vi "refocusAndReposition.vi"() -> ()   [LabVIEW 2022 SP3]
panel:
  in  "Point of Interest - y":dbl
  in  "Point of Interest - x":dbl
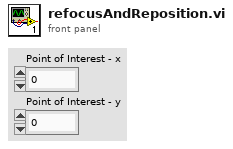
[diagram p1: front panel]
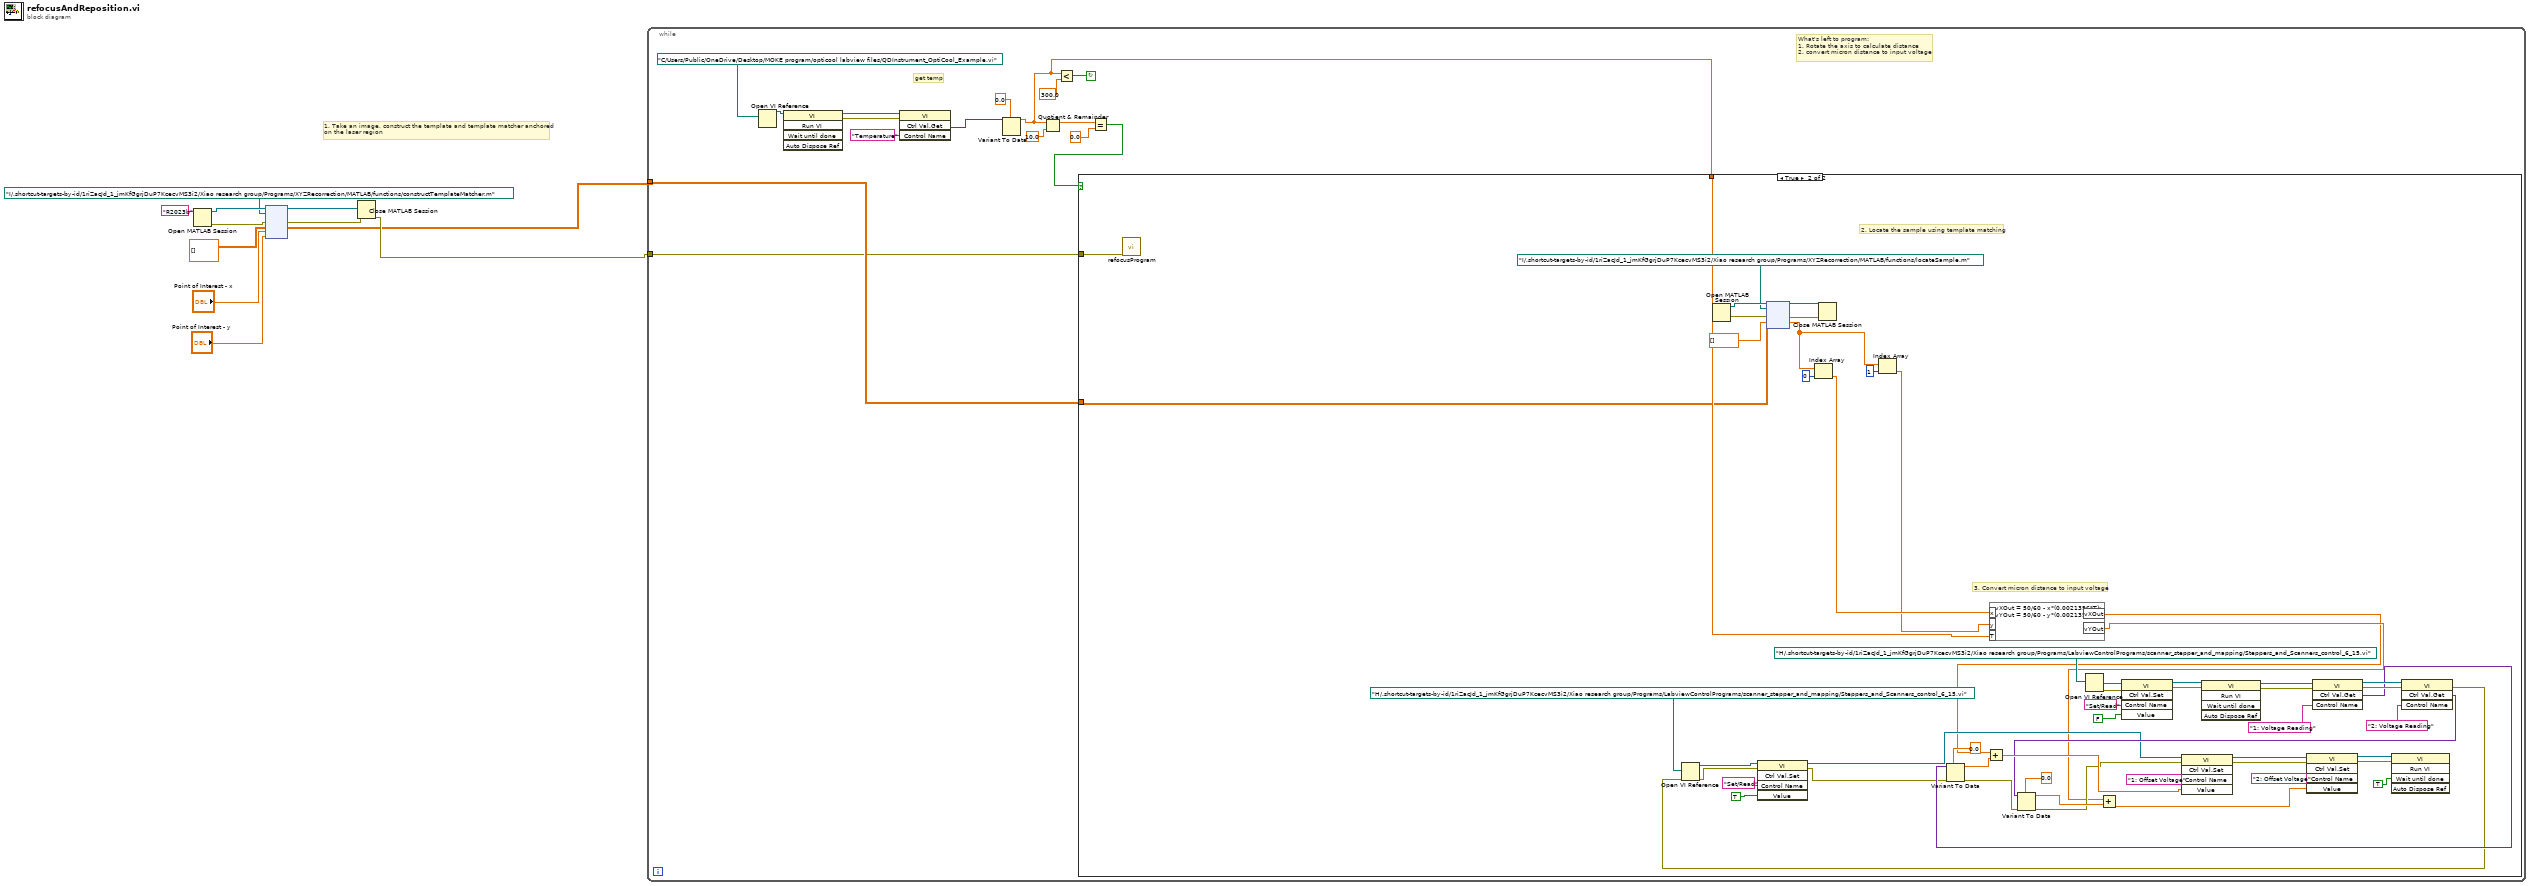
[diagram p0: block diagram]
diagram:
  # "1. Take an image, construct the template and template matcher anchored\non the laser region"
  n1 = Open MATLAB Session(0:"R2023b" ("release name")) -> (8:w11:refnum<k37>, 11:w10:errorcluster)  [unwired: 1 in]
  n2 = node(w11, path "I:/.shortcut-targets-by-id/1riZacJd_1_jmKfGgrjDuP7KcecvMS3i2/Xiao research group/Programs/XYZRecorrection/MATLAB/functions/constructTemplateMatcher.m" ("source file path"), w10, dbl[][] [], "Point of Interest - x", "Point of Interest - y") -> (w5:refnum<k37>, w4:errorcluster, w1:dbl[][])  [unwired: 3 in, 2 out]
  n3 = Close MATLAB Session(0:w5, 3:w4) -> (11:w2:errorcluster)
  n4 = while {
    tunnel: w1 -> [w14]
    tunnel: w2 -> [w13]
    stop <- w20 continue-if-true
    # "get temp"
    # "What's left to program:\n1. Rotate the axis to calculate distance\n2. convert micron distance to input voltage"
    n5 = Open VI Reference(vi path=path "C:/Users/Public/OneDrive/Desktop/MOKE program/opticool labview files/QDInstrument_OptiCool_Example.vi") -> (vi reference=w24:refnum<vi>)  [unwired: 5 in, 1 out]
    n6 = invoke class="VI" method="Run VI"(reference=w24) -> (reference out=w25:refnum<vi>, error out=w26:errorcluster)  [unwired: 4 in, 3 out]
    n7 = invoke class="VI" method="Ctrl Val.Get"(reference=w25, error in=w26, "Control Name"="Temperature") -> ("Get Control Value Variant"=w27:variant)  [unwired: 1 in, 3 out]
    n8 = Variant To Data(type=0.0, Variant=w27) -> (data=w12:dbl)  [unwired: 1 in, 1 out]
    n9 = Quotient & Remainder(x=w12, y=10.0) -> (x-y*floor(x/y)=w17:dbl)  [unwired: 1 out]
    n10 = Less?(x=w12, y=300.0) -> (x < y?=w20:bool)
    n11 = Equal?(x=w17, y=0.0) -> (x = y?=w15:bool)
    n12 = case shown="True" w15 {
      tunnel: w14 -> [_ w70]
      tunnel: w13 -> [_ w81]
      tunnel: w12 -> [_ w80]
      frame False {
      }
      frame True {
        # "3. Convert micron distance to input voltage"
        # "2. Locate the sample using template matching"
        n13 = call "refocusProgram.vi"("error in (no error)"=w81) -> ()  [unwired: 11 in]
        n14 = Open MATLAB Session() -> (8:w79:refnum<k37>, 11:w76:errorcluster)  [unwired: 2 in]
        n15 = node(w79, path "I:/.shortcut-targets-by-id/1riZacJd_1_jmKfGgrjDuP7KcecvMS3i2/Xiao research group/Programs/XYZRecorrection/MATLAB/functions/locateSample.m" ("source file path"), w76, dbl[] [], w70) -> (w78:refnum<k37>, w77:errorcluster, w72:dbl[])  [unwired: 2 in, 2 out]
        n16 = Index Array(array=w72, index=0 ("index (row)")) -> (element=w69:dbl)
        n17 = Close MATLAB Session(0:w78, 3:w77) -> ()  [unwired: 1 out]
        n18 = Index Array(array=w72, index=1 ("index (row)")) -> (element=w68:dbl)
        n19 = formula code="vXOut = 50/60 - x*(0.0021396*T);\nvYOut = 50/60 - y*(0.0021396*T);"("x"=w69, "y"=w68, "T"=w80) -> ("vXOut"=w28:dbl, "vYOut"=w29:dbl)
        n20 = Open VI Reference(vi path=path "H:/.shortcut-targets-by-id/1riZacJd_1_jmKfGgrjDuP7KcecvMS3i2/Xiao research group/Programs/LabviewControlPrograms/scanner_stepper_and_mapping/Steppers_and_Scanners_control_6_15.vi") -> (vi reference=w59:refnum<vi>, error out=w58:errorcluster)  [unwired: 5 in]
        n21 = invoke class="VI" method="Ctrl Val.Set"(reference=w59, error in=w58, "Control Name"="Set/Read", "Value"=FALSE ("Wait Until Done")) -> (reference out=w57:refnum<vi>, error out=w56:errorcluster)  [unwired: 1 in, 3 out]
        n22 = invoke class="VI" method="Run VI"(reference=w57, error in=w56) -> (reference out=w53:refnum<vi>, error out=w52:errorcluster)  [unwired: 3 in, 3 out]
        n23 = invoke class="VI" method="Ctrl Val.Get"(reference=w53, error in=w52, "Control Name"="1: Voltage Reading") -> (reference out=w50:refnum<vi>, error out=w49:errorcluster, "Get Control Value Variant"=w47:variant)  [unwired: 1 in, 1 out]
        n24 = invoke class="VI" method="Ctrl Val.Get"(reference=w50, error in=w49, "Control Name"="2: Voltage Reading") -> (error out=w36:errorcluster, "Get Control Value Variant"=w40:variant)  [unwired: 1 in, 2 out]
        n25 = Open VI Reference(vi path=path "H:/.shortcut-targets-by-id/1riZacJd_1_jmKfGgrjDuP7KcecvMS3i2/Xiao research group/Programs/LabviewControlPrograms/scanner_stepper_and_mapping/Steppers_and_Scanners_control_6_15.vi", error in (no error)=w36) -> (vi reference=w33:refnum<vi>, error out=w32:errorcluster)  [unwired: 4 in]
        n26 = invoke class="VI" method="Ctrl Val.Set"(reference=w33, error in=w32, "Control Name"="Set/Read", "Value"=TRUE ("Wait Until Done")) -> (reference out=w31:refnum<vi>, error out=w30:errorcluster)  [unwired: 1 in, 3 out]
        n27 = Variant To Data(error in=w30, type=0.0, Variant=w47) -> (data=w45:dbl, error out=w41:errorcluster)
        n28 = Add(x=w28, y=w45) -> (x+y=w44:dbl)
        n29 = Variant To Data(error in=w41, type=0.0, Variant=w40) -> (data=w42:dbl, error out=w39:errorcluster)
        n30 = Add(x=w29, y=w42) -> (x+y=w38:dbl)
        n31 = invoke class="VI" method="Ctrl Val.Set"(reference=w31, error in=w39, "Control Name"="1: Offset Voltage", "Value"=w44) -> (reference out=w64:refnum<vi>, error out=w65:errorcluster)  [unwired: 1 in, 3 out]
        n32 = invoke class="VI" method="Ctrl Val.Set"(reference=w64, error in=w65, "Control Name"="2: Offset Voltage", "Value"=w38) -> (reference out=w66:refnum<vi>, error out=w67:errorcluster)  [unwired: 1 in, 3 out]
        n33 = invoke class="VI" method="Run VI"(reference=w66, error in=w67, "Wait until done"=TRUE ("Wait Until Done")) -> ()  [unwired: 2 in, 5 out]
      }
    }
  }
